vi "RTS Save Station.vi"(6 "Station Number":u8=1 min=1 max=8 step=1, 7 "Custom Saved Titles":string[][](array[string]), 8 "error in (no error)":errorcluster, 10 "RTS Config Setup Save Loop":T1, 11 "TDMS Data Save Loop":T10) -> (0 "error out":errorcluster, 2 "RTS Config Setup Save Loop Out":T1, 3 "CSV Data Save Output":T10)   [LabVIEW 2016]
uses:
  Type Definitions/RTS TDMS Filename Locations.ctl
  Type Definitions/RTS Save References.ctl
  Type Definitions/RTS Configuration Setup.ctl
  Type Definitions/RTS Wago Config.ctl
  Type Definitions/RTS APLUS Config.ctl
  Type Definitions/RTS Yokogawa MX Config.ctl
  Type Definitions/RTS Replay Server Control.ctl
  Type Definitions/RTS Server Configuration.ctl
  Type Definitions/RTS Station Settions TCP Comms.ctl
  Type Definitions/RTS Chamber Save Status.ctl
  Type Definitions/RTS Test Pattern.ctl
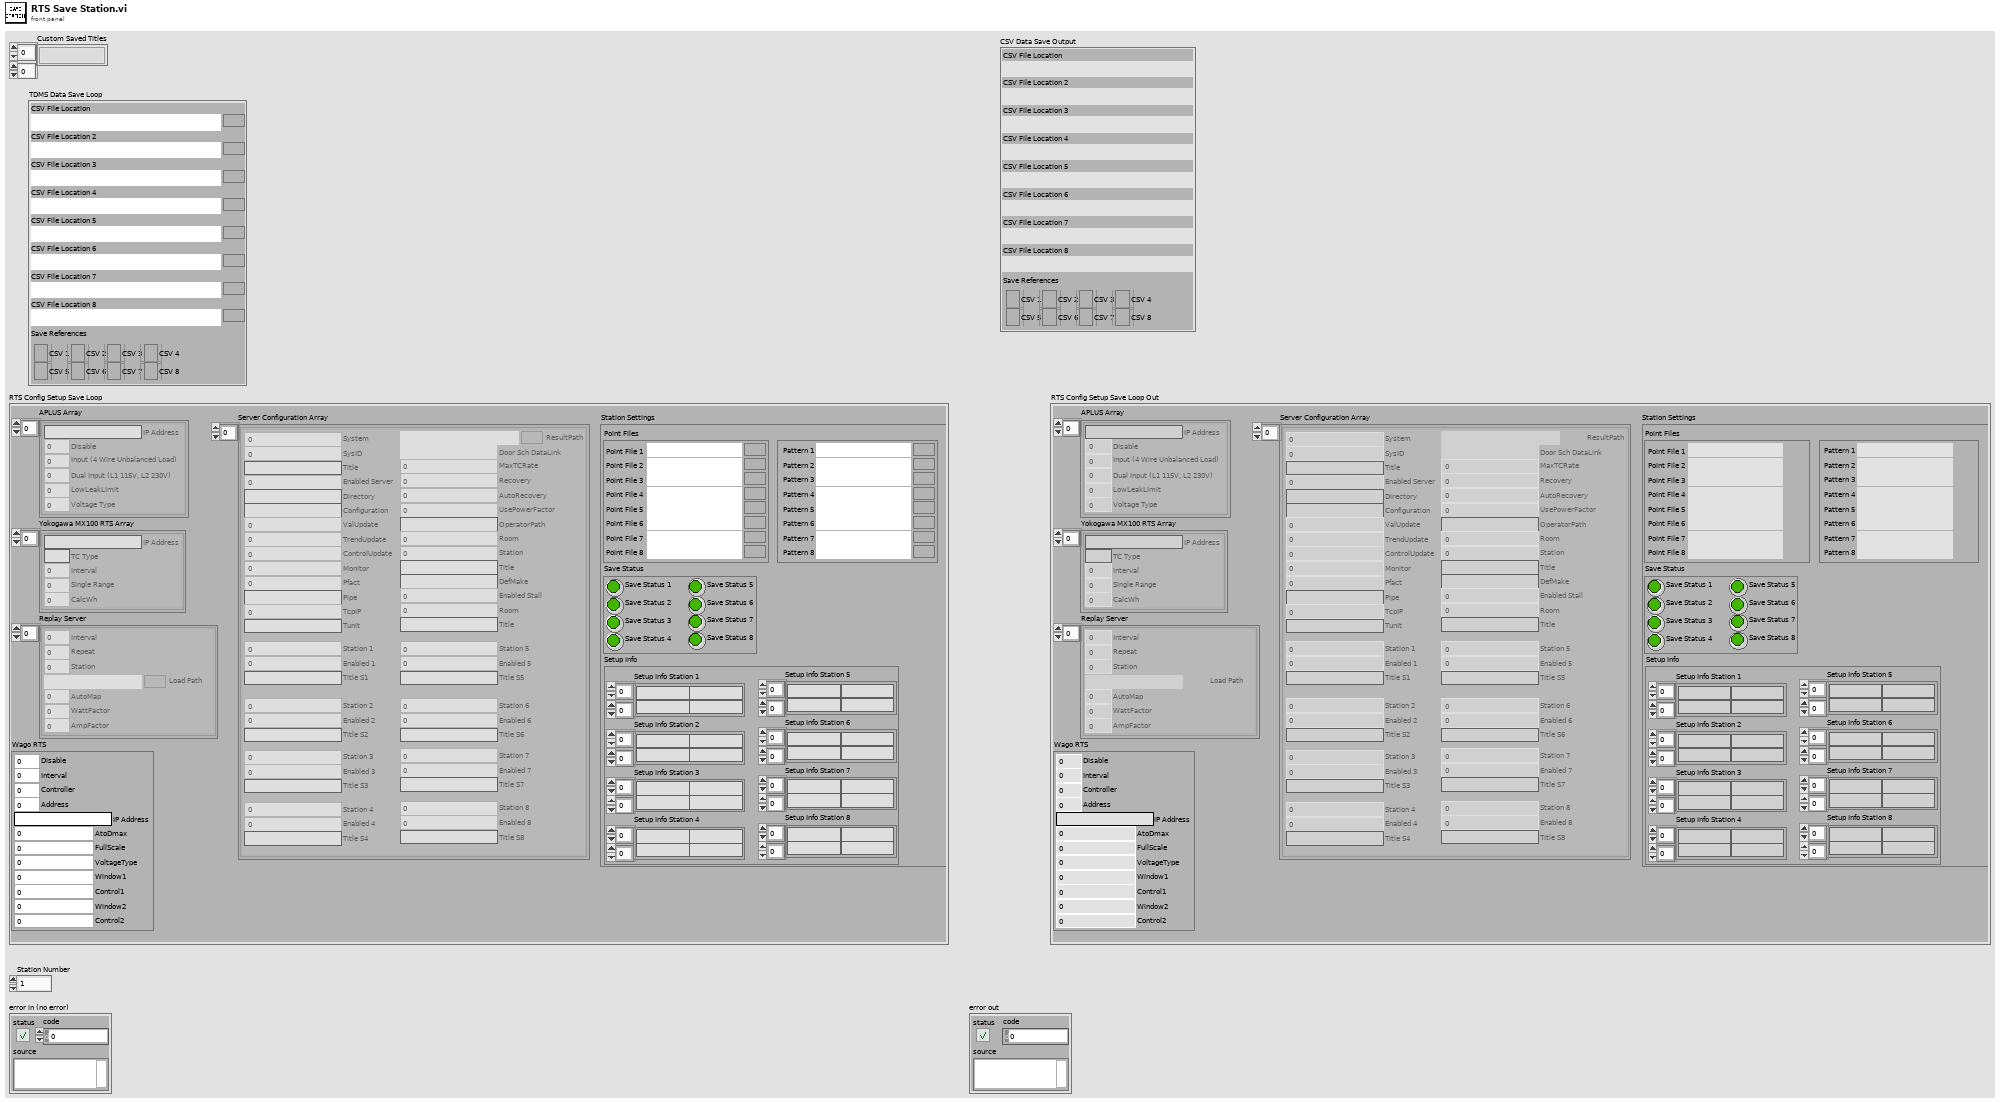
[diagram p1: front panel]
types:
  T1 = typedef "RTS Configuration Setup.ctl" = cluster{"Wago RTS":T2, "APLUS Array":T3[], "Yokogawa MX100 RTS Array":T4[], "Replay Server":T5[], "Server Configuration Array":T6[], "Station Settings":T7}
  T2 = typedef "RTS Wago Config.ctl" = cluster{"Disable":u16, "Interval":u16, "Controller":u16, "Address":u16, "IP Address":string, "AtoDmax":u16, "FullScale":u16, "VoltageType":u16, "Window1":u16, "Control1":u16, "Window2":u16, "Control2":u16}
  T3 = typedef "RTS APLUS Config.ctl" = cluster{"Disable":u16, "IP Address":string, "Input (4 Wire Unbalanced Load)":u16, "Dual Input (L1 115V, L2 230V)":u16, "LowLeakLimit":dbl, "Voltage Type":u16}
  T4 = typedef "RTS Yokogawa MX Config.ctl" = cluster{"IP Address":string, "TC Type":string, "Interval":u16, "Single Range":u16, "CalcWh":u16}
  T5 = typedef "RTS Replay Server Control.ctl" = cluster{"Interval":i16, "Repeat":u16, "Station":u16, "Load Path":path, "AutoMap":u16, "WattFactor":dbl, "AmpFactor":dbl}
  T6 = typedef "RTS Server Configuration.ctl" = cluster{"System":u16, "SysID":u16, "Title":string, "Enabled Server":u16, "Directory":string, "Configuration":string, "ValUpdate":u16, "TrendUpdate":u16, "ControlUpdate":u16, "Monitor":u16, "Pfact":u16, "Pipe":string, "TcpIP":u16, "Tunit":string, "ResultPath":path, "Door Sch DataLink":path, "MaxTCRate":u16, "Recovery":u16, "AutoRecovery":u16, "UsePowerFactor":u16, "OperatorPath":string, "Room":u16, "Station":u16, "Title":string, "DefMake":string, "Enabled Stall":u16, "Room":u16, "Title":string, "Station 1":u16, "Enabled 1":u16, "Station 2":u16, "Enabled 2":u16, "Station 3":u16, "Enabled 3":u16, "Station 4":u16, "Enabled 4":u16, "Station 5":u16, "Enabled 5":u16, "Station 6":u16, "Enabled 6":u16, "Station 7":u16, "Enabled 7":u16, "Station 8":u16, "Enabled 8":u16, "Title S1":string, "Title S2":string, "Title S3":string, "Title S5":string, "Title S6":string, "Title S7":string, "Title S8":string, "Title S4":string}
  T7 = typedef "RTS Station Settions TCP Comms.ctl" = cluster{"Point Files":cluster{"Point File 1":path, "Point File 2":path, "Point File 3":path, "Point File 4":path, "Point File 5":path, "Point File 6":path, "Point File 7":path, "Point File 8":path}, "Save Status":T8, "Setup Info":cluster{"Setup Info Station 1":string[][], "Setup Info Station 2":string[][], "Setup Info Station 3":string[][], "Setup Info Station 4":string[][], "Setup Info Station 5":string[][], "Setup Info Station 6":string[][], "Setup Info Station 7":string[][], "Setup Info Station 8":string[][]}, "Chamber Test Pattern":T9}
  T8 = typedef "RTS Chamber Save Status.ctl" = cluster{"Save Status 1":bool, "Save Status 2":bool, "Save Status 3":bool, "Save Status 4":bool, "Save Status 5":bool, "Save Status 6":bool, "Save Status 7":bool, "Save Status 8":bool}
  T9 = typedef "RTS Test Pattern.ctl" = cluster{" Pattern 1":path, "Pattern 2":path, "Pattern 3":path, "Pattern 4":path, "Pattern 5":path, "Pattern 6":path, "Pattern 7":path, "Pattern 8":path}
  T10 = typedef "RTS TDMS Filename Locations.ctl" = cluster{"CSV File Location":path, "CSV File Location 2":path, "CSV File Location 3":path, "CSV File Location 4":path, "CSV File Location 5":path, "CSV File Location 6":path, "CSV File Location 7":path, "CSV File Location 8":path, "Save References":T11}
  T11 = typedef "RTS Save References.ctl" = cluster{"CSV 1":refnum<file>, "CSV 2":refnum<file>, "CSV 3":refnum<file>, "CSV 4":refnum<file>, "CSV 5":refnum<file>, "CSV 6":refnum<file>, "CSV 7":refnum<file>, "CSV 8":refnum<file>}
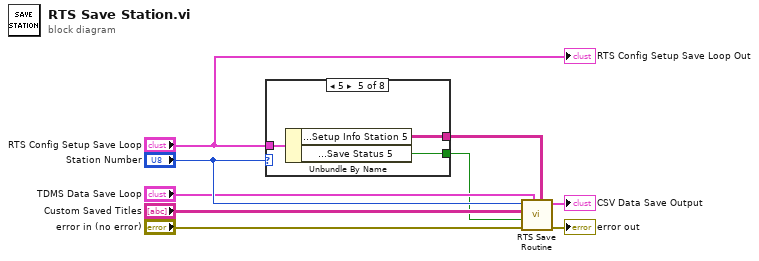
[diagram p0: block diagram]
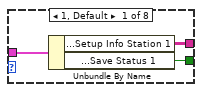
[diagram p2: hidden frame]
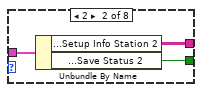
[diagram p3: hidden frame]
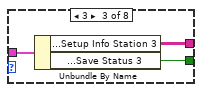
[diagram p4: hidden frame]
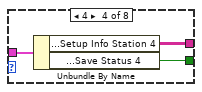
[diagram p5: hidden frame]
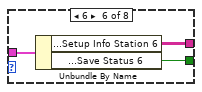
[diagram p6: hidden frame]
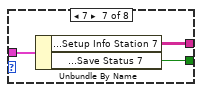
[diagram p7: hidden frame]
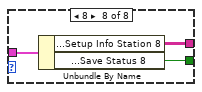
[diagram p8: hidden frame]
diagram:
  n1 = case shown="5" "Station Number" {
    tunnel: "RTS Config Setup Save Loop" -> [w12 w15 w18 w21 w24 w27 w30 w33]
    tunnel: [w10 w13 w16 w19 w22 w25 w28 w31] -> w5
    tunnel: [w11 w14 w17 w20 w23 w26 w29 w32] -> w4
    frame 1, Default {
      n2 = Unbundle By Name(w12) -> ("Station Settings.Setup Info.Setup Info Station 1"=w11:string[][], "Station Settings.Save Status.Save Status 1"=w10:bool)
    }
    frame 2 {
      n3 = Unbundle By Name(w15) -> ("Station Settings.Setup Info.Setup Info Station 2"=w14:string[][], "Station Settings.Save Status.Save Status 2"=w13:bool)
    }
    frame 3 {
      n4 = Unbundle By Name(w18) -> ("Station Settings.Setup Info.Setup Info Station 3"=w17:string[][], "Station Settings.Save Status.Save Status 3"=w16:bool)
    }
    frame 4 {
      n5 = Unbundle By Name(w21) -> ("Station Settings.Setup Info.Setup Info Station 4"=w20:string[][], "Station Settings.Save Status.Save Status 4"=w19:bool)
    }
    frame 5 {
      n6 = Unbundle By Name(w24) -> ("Station Settings.Setup Info.Setup Info Station 5"=w23:string[][], "Station Settings.Save Status.Save Status 5"=w22:bool)
    }
    frame 6 {
      n7 = Unbundle By Name(w27) -> ("Station Settings.Setup Info.Setup Info Station 6"=w26:string[][], "Station Settings.Save Status.Save Status 6"=w25:bool)
    }
    frame 7 {
      n8 = Unbundle By Name(w30) -> ("Station Settings.Setup Info.Setup Info Station 7"=w29:string[][], "Station Settings.Save Status.Save Status 7"=w28:bool)
    }
    frame 8 {
      n9 = Unbundle By Name(w33) -> ("Station Settings.Setup Info.Setup Info Station 8"=w32:string[][], "Station Settings.Save Status.Save Status 8"=w31:bool)
    }
  }
  n10 = call "RTS Save Routine.vi"("Setup Info Station 8"=w4, "TDMS Data Save Input"="TDMS Data Save Loop", "error in (no error)"="error in (no error)", "Save Status 8"=w5, "Custom Saved Titles"="Custom Saved Titles", "Station Number"="Station Number") -> ("error out"=→"error out":errorcluster, "CSV Data Save Output"=→"CSV Data Save Output":T10)  [unwired: 4 in]
  "RTS Config Setup Save Loop Out" <- "RTS Config Setup Save Loop"
